vi "PCOValidFirewireLines.vi"(2 "wYResAct":u32, 3 "wXResAct":u32=1 min=1 max=32000) -> (0 "ValidBytes":u32, 1 "Y-Lines needed":i32)   [LabVIEW 2011]
panel:
  # "SDK page 135\nIn case of using FireWire interface and if the user allocates external image buffer, the size of the \nbuffer must to be a multiple of 4096 (0x1000) + 8192 bytes."
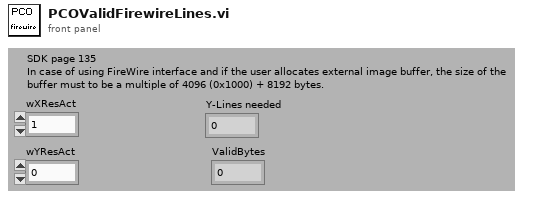
[diagram p1: front panel]
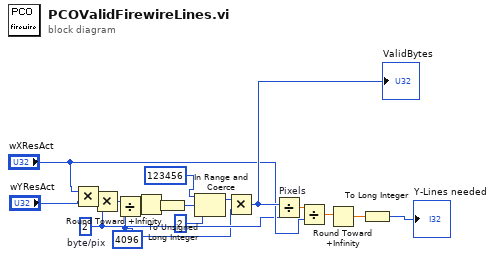
[diagram p0: block diagram]
diagram:
  w11 = u32 2  # byte/pix
  w10 = u32 4096 ("y")
  n1 = Multiply(x="wXResAct", y="wYResAct") -> (x*y=w8:u32)
  n2 = Multiply(x=w8, y=w11) -> (x*y=w9:u32)
  n3 = Divide(x=w9, y=w10) -> (x/y=w1:dbl)
  n4 = Round Toward +Infinity(x=w1) -> (ceil(x): smallest int >= x=w2:dbl)
  n5 = To Unsigned Long Integer(number=w2) -> (unsigned 32bit integer=w5:u32)
  n6 = In Range and Coerce(upper limit=u32 123456, x=w5, lower limit=u32 2) -> (coerced(x)=w4:u32)  [unwired: 1 out]
  n7 = Multiply(x=w4, y=w10) -> (x*y=w16:u32)
  "ValidBytes" <- w16
  n8 = Divide "Pixels"(x=w16, y=w11) -> (x/y=w12:dbl)
  n9 = Divide(x=w12, y="wXResAct") -> (x/y=w14:dbl)
  n10 = Round Toward +Infinity(x=w14) -> (ceil(x): smallest int >= x=w15:dbl)
  n11 = To Long Integer(number=w15) -> (32bit integer=→"Y-Lines needed":i32)
